vi "Check Pressure Stabilize.vi"(10 "Numeric in":sgl, 11 "Test Pressure":i32) -> (3 "Numeric out":sgl)   [LabVIEW 2020]
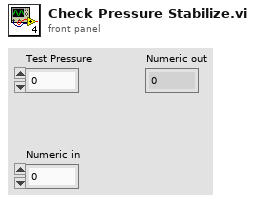
[diagram p1: front panel]
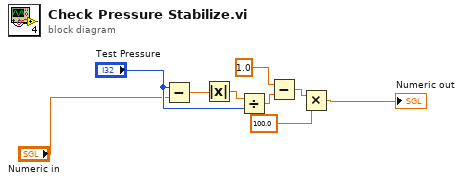
[diagram p0: block diagram]
diagram:
  n1 = Subtract(x="Test Pressure", y="Numeric in") -> (x-y=w2:sgl)
  n2 = Absolute Value(x=w2) -> (abs(x)=w3:sgl)
  n3 = Divide(x=w3, y="Test Pressure") -> (x/y=w5:sgl)
  n4 = Subtract(x=sgl 1.0, y=w5) -> (x-y=w7:sgl)
  n5 = Multiply(x=w7, y=sgl 100.0) -> (x*y=→"Numeric out":sgl)
